vi "Format Call Chain.vi"(11 "Call Chain Array":string[](array[string])) -> (3 "Calling VI":string)   [LabVIEW 2019, in "Application.lvclass"]
uses:
  Application.lvclass
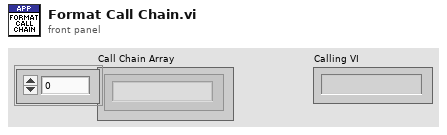
[diagram p1: front panel]
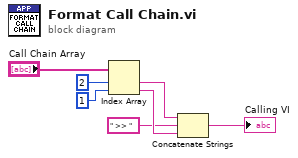
[diagram p0: block diagram]
diagram:
  n1 = Index Array(array="Call Chain Array", index #1=2 ("index"), index #2=1 ("index")) -> (element #1=w5:string, element #2=w4:string)
  n2 = Concatenate Strings(w5, " >> " ("string"), w4) -> (→"Calling VI":string)
